vi "SetDC Offset.vi"(6 "DC offset [V]":dbl caption="DC offset", 8 "error in (no error)":errorcluster, 9 "channel":i32, 10 "Fpga input":T1, 11 "Scope5761 in":refnum<class "Scope5761.lvclass">) -> (0 "error out":errorcluster, 3 "Scope5761 out":refnum<class "Scope5761.lvclass">)   [LabVIEW 2013, in "Scope5761.lvclass"]
uses:
  Scope5761.lvclass
  fpga ID.ctl
  Scope5761.lvclass/Scope5761.ctl
  FPGA/fpga_settings.ctl
  <vilib>/rvi/FXPMathLib/FxpInterpret/XNode/nifxpmath_Interpret.xnode
  FpgaRef/FpgaRefBase/FpgaRefBase.lvclass
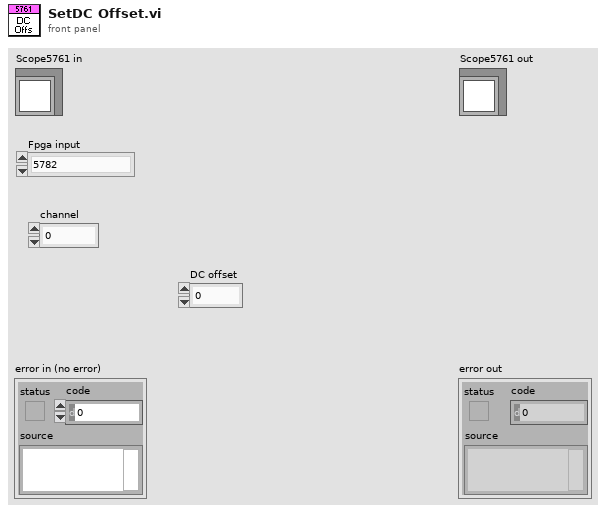
[diagram p1: front panel]
types:
  T1 = typedef "Scope5761.lvclass/fpga ID.ctl" = enum16{"5782", "5761 - 1", "5761 - 2"}
  T2 = typedef "fpga_settings.ctl" = enum16{"Feedback Enable", "New FIR coeffs", "FIR shift", "Enable filter", "Set Downsample", "Downsample", "CIC Gain", "Record length", "Trigger samples", "Quiet time", "a_am", "b_am", "Use fixed delay", "fixed sin_fi", "fixed cos_fi", "Ki*Tau", "Kp", "Kd_Tau", "Fi_start", "Fi_delta", "DC_offs 0", "DC_offs 1", "DC_offs 2", "DC_offs 3", "Ki*Tau am", "Kp am", "Kd_Tau am", "Feedback AM", "Trigger delay", "Feedback delay", "Setpoint enable", "Beam enable", "Samples to acquire", "Cavity Enable"}
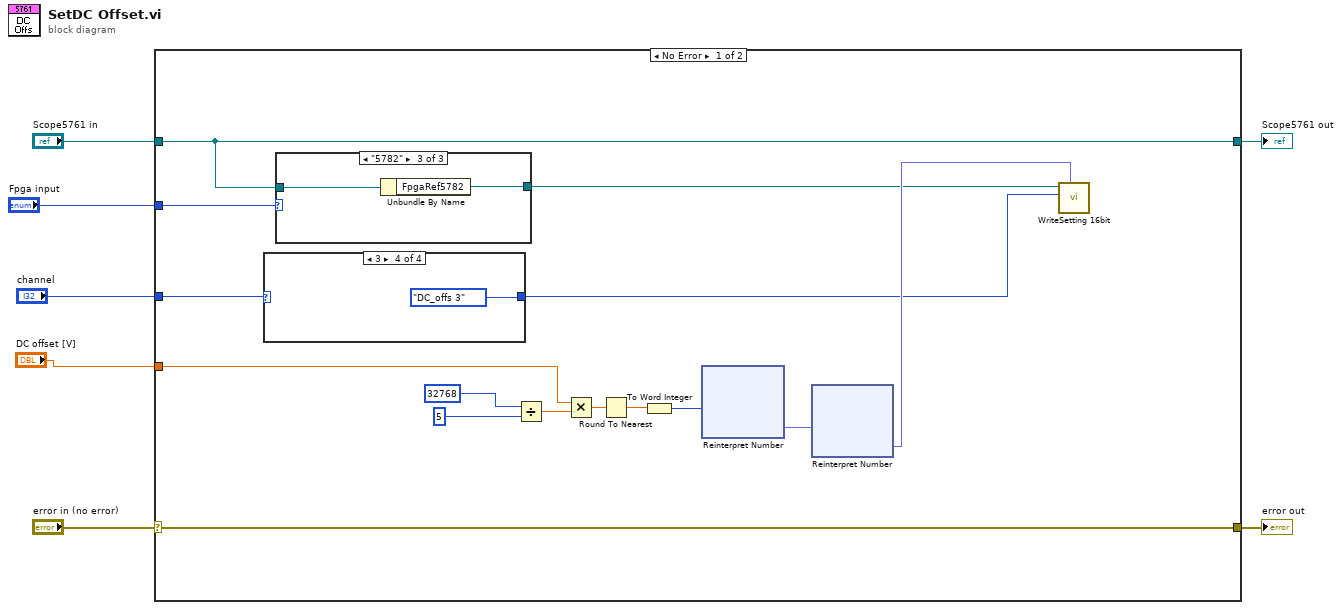
[diagram p0: block diagram]
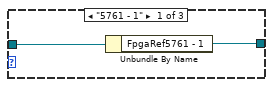
[diagram p2: hidden frame]
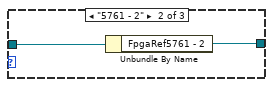
[diagram p3: hidden frame]
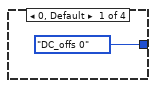
[diagram p4: hidden frame]
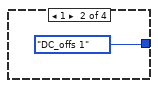
[diagram p5: hidden frame]
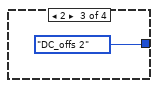
[diagram p6: hidden frame]
diagram:
  n1 = case shown="No Error" "error in (no error)" {
    selector: "error in (no error)" -> [w22 w34]
    tunnel: [w22 w34] -> w6
    tunnel: [w10 w33] -> w4
    tunnel: "Scope5761 in" -> [w10 w33]
    tunnel: "DC offset [V]" -> [w14 _]
    tunnel: "channel" -> [w13 _]
    tunnel: "Fpga input" -> [w11 _]
    frame No Error {
      n2 = case shown="3" w13 {
        tunnel: [fpga_settings."DC_offs 0" ("FPGA Setting") fpga_settings."DC_offs 1" ("FPGA Setting") fpga_settings."DC_offs 2" ("FPGA Setting") fpga_settings."DC_offs 3" ("FPGA Setting")] -> w8
        frame 0, Default {
        }
        frame 1 {
        }
        frame 2 {
        }
        frame 3 {
        }
      }
      n3 = case shown="\"5782\"" w11 {
        tunnel: w10 -> [w24 w26 w28]
        tunnel: [w23 w25 w27] -> w9
        frame "5761 - 1" {
          n4 = Unbundle By Name(w24) -> ("FpgaRef5761 - 1"=w23:refnum<class "FpgaRef5761.lvclass">)
        }
        frame "5761 - 2" {
          n5 = Unbundle By Name(w26) -> ("FpgaRef5761 - 2"=w25:refnum<class "FpgaRef5761.lvclass">)
        }
        frame "5782" {
          n6 = Unbundle By Name(w28) -> ("FpgaRef5782"=w27:refnum<class "FpgaRef5782.lvclass">)
        }
      }
      n7 = Divide(x=32768, y=5) -> (x/y=w19:dbl)
      n8 = Multiply(x=w14, y=w19) -> (x*y=w18:dbl)
      n9 = Round To Nearest(number=w18) -> (nearest integer value=w17:dbl)
      n10 = To Word Integer(number=w17) -> (16bit integer=w16:i16)
      n11 = xnode "Reinterpret Number"("x"=w16) -> ("y"=w15:fxp<+/-,16,14>)
      n12 = xnode "Reinterpret Number"("x"=w15) -> ("y"=w12:fxp<+,16,16>)
      n13 = call "WriteSetting 16bit.vi"("value"=w12, "FPGA Setting"=w8, "FpgaRefBase in"=w9) -> ()  [unwired: 7 in, 2 out]
    }
    frame Error {
    }
  }
  "error out" <- w6
  "Scope5761 out" <- w4
